vi "Hindbrain.vi"() -> ()   [LabVIEW 2012]
doc: "Hindbrain_RobotBrainExample. This VI is an example of the Hindbrain layer of the Olin Robot Architecture. It collects all SENSE data and sends it up three neural clusters to the Midbrain and accepts one ACT cluster from Midbrain to drive all robot actuators. \nVI also contains a simple robot simulation to allow control code development"
uses:
  GlobalACT.vi
  WindDir.vi
  WindSpeed.vi
  G_Boat Speed.vi
  GlobalWhatAroundMe.vi
  GlobalWhereAmI.vi
  GlobalHowAmI.vi
panel:
  out "WhereSensor":T1
  out "Act Command":cluster{"Velocity":dbl, "Direction":dbl}
  out "Act":bool
  out "How?":bool
  out "What?":bool
  in  "stop":bool
  out "Where":bool
  out "HowAmI?":cluster{"T":dbl, "Battery":dbl, "Temp":dbl}
  out "WhatAroundMe?":cluster{"T":dbl, "Range":dbl, "Bearing":dbl}[](array[cluster])
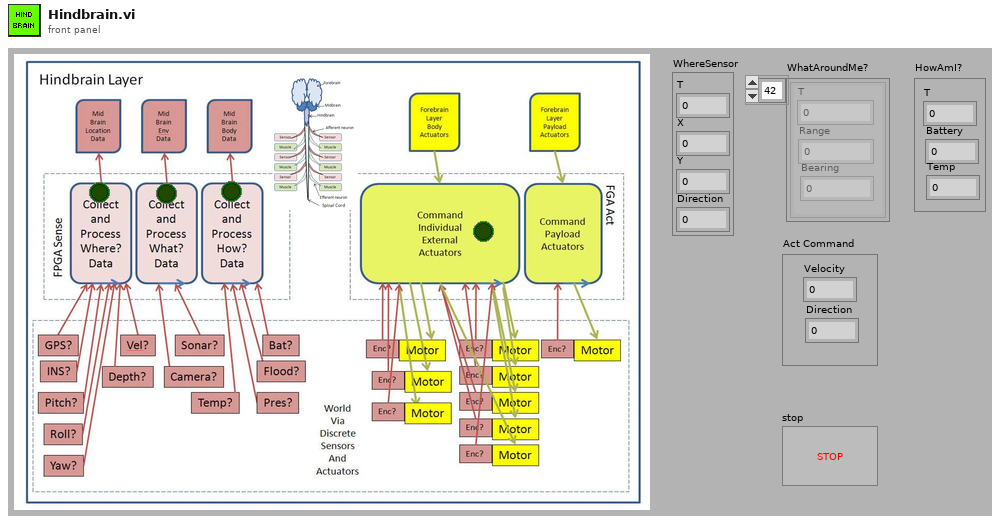
[diagram p1: front panel]
types:
  T1 = cluster{"T":dbl, "X":dbl, "Y":dbl, "Direction":dbl}
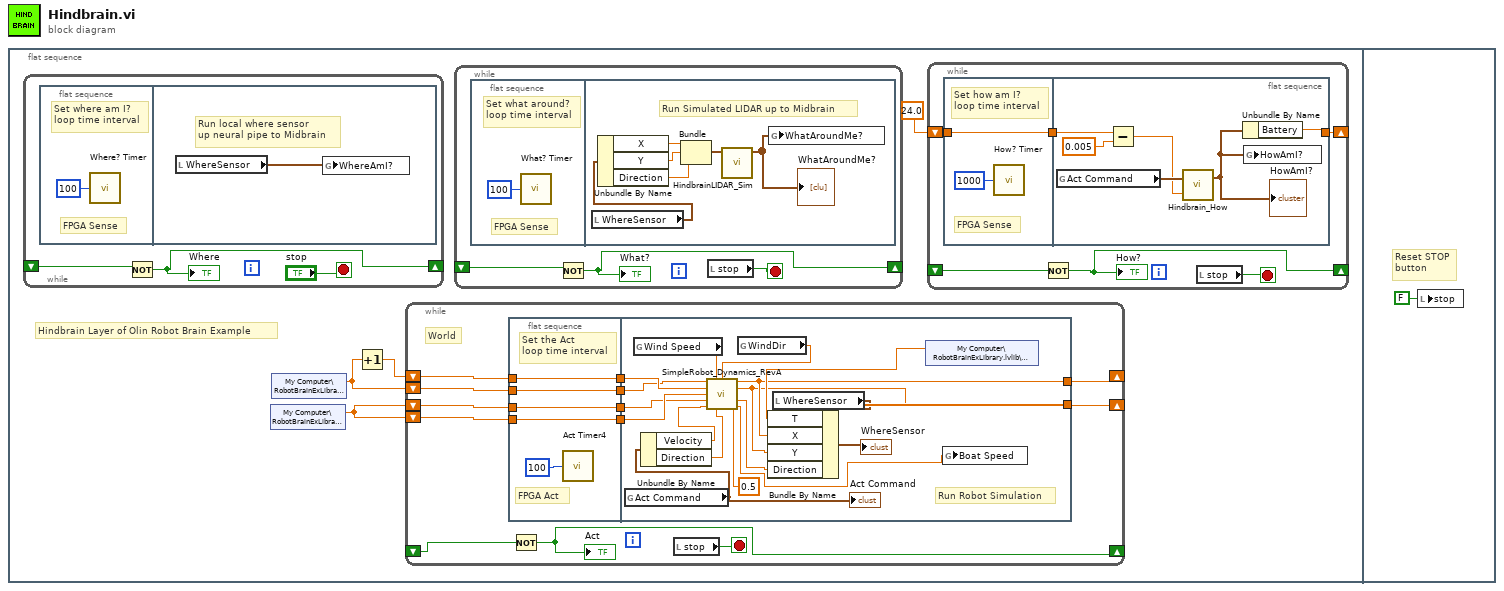
[diagram p0: block diagram]
diagram:
  n1 = flat-sequence {
    frame #0 {
      # "Hindbrain Layer of Olin Robot Brain Example"
      n2 = while {
        shift-right: [w64] -> _
        shift-left: _ -> [w65]
        stop <- "stop" stop-if-true
        n3 = flat-sequence {
          frame #0 {
            # "FPGA Sense"
            # "Set where am I?\nloop time interval"
            n4 = call "Where? Timer"("Count(mSec)"=u32 100) -> ()  [unwired: 1 out]
          }
          frame #1 {
            # "Run local where sensor\nup neural pipe to Midbrain"
            n5 = local read "WhereSensor"() -> (w68:T1)
            n6 = global write "GlobalWhereAmI.vi" "WhereAmI?"(w68) -> ()
          }
        }
        n7 = Not(x=w65) -> (.not. x?=w64:bool)
        "Where" <- w64
      }
      n8 = shared-variable "My Computer\\RobotBrainExLibrary.lvlib\\Ystart"() -> (w3:dbl)  [unwired: 1 in, 1 out]
      n9 = shared-variable "My Computer\\RobotBrainExLibrary.lvlib\\Xstart"() -> (w2:dbl)  [unwired: 1 in, 1 out]
      n10 = Increment(x=w2) -> (x+1=w1:dbl)
      n11 = while {
        shift-right: [w16] -> _
        shift-left: _ -> [w17]
        shift-right: [w6] -> _
        shift-left: w1 -> [w13]
        shift-left: w2 -> [w11]
        shift-right: [w5] -> _
        shift-left: w3 -> [w9]
        shift-left: w3 -> [w7]
        stop <- w15 stop-if-true
        # "World"
        n12 = flat-sequence {
          tunnel: [w21] -> w14
          tunnel: w13 -> [w21]
          tunnel: [w20] -> w12
          tunnel: w11 -> [w20]
          tunnel: [w19] -> w10
          tunnel: w9 -> [w19]
          tunnel: [w18] -> w8
          tunnel: w7 -> [w18]
          tunnel: w14 -> [w29]
          tunnel: [w34] -> w6
          tunnel: w12 -> [w28]
          tunnel: w10 -> [w26]
          tunnel: [w33] -> w5
          tunnel: w8 -> [w27]
          frame #0 {
            # "FPGA Act"
            # "Set the Act\nloop time interval"
            n13 = call "Act Timer4"("Count(mSec)"=u32 100) -> ()  [unwired: 1 out]
          }
          frame #1 {
            # "Run Robot Simulation"
            n14 = global read "GlobalACT.vi" "Act Command"() -> (w39:cluster{"Velocity":dbl, "Direction":dbl})
            "Act Command" <- w39
            n15 = global read "WindSpeed.vi" "Wind Speed"() -> (w25:dbl)
            n16 = Unbundle By Name(w39) -> ("Velocity"=w38:dbl, "Direction"=w37:dbl)
            n17 = global read "WindDir.vi" "WindDir"() -> (w24:dbl)
            n18 = call "SimpleRobot_Dynamics_RevA.vi"("x0"=w28, "Wind Speed"=w25, "Wind Direction"=w24, "x1"=w29, "y0"=w27, "y1"=w26, "Velocity"=w38, "Direction"=w37, "DeltaT (timestep)"=0.5) -> ("x 2"=w34:dbl, "y 2"=w33:dbl, "Direction 2"=w32:dbl, "Boat Velocity Out"=w23:dbl)  [unwired: 3 in]
            n19 = local read "WhereSensor"() -> (w30:T1)
            n20 = shared-variable "My Computer\\RobotBrainExLibrary.lvlib\\MissionTime"() -> (w35:dbl)  [unwired: 1 in, 1 out]
            n21 = Bundle By Name(cluster=w30, "T"=w35, "X"=w34, "Y"=w33, "Direction"=w32) -> (→"WhereSensor":T1)
            n22 = global write "G_Boat Speed.vi" "Boat Speed"(w23) -> ()
          }
        }
        n23 = Not(x=w17) -> (.not. x?=w16:bool)
        "Act" <- w16
        n24 = local read "stop"() -> (w15:bool)
      }
      n25 = while {
        shift-right: [w55] -> _
        shift-left: _ -> [w56]
        stop <- w54 stop-if-true
        n26 = flat-sequence {
          frame #0 {
            # "FPGA Sense"
            # "Set what around?\nloop time interval"
            n27 = call "What? Timer"("Count(mSec)"=u32 100) -> ()  [unwired: 1 out]
          }
          frame #1 {
            # "Run Simulated LIDAR up to Midbrain"
            n28 = local read "WhereSensor"() -> (w62:T1)
            n29 = Unbundle By Name(w62) -> ("X"=w60:dbl, "Y"=w59:dbl, "Direction"=w58:dbl)
            n30 = Bundle("X"=w60, "Y"=w59, "Direction"=w58) -> (w61:cluster{"X":dbl, "Y":dbl, "Direction":dbl})  [unwired: 1 in]
            n31 = call "HindbrainLIDAR_Sim.vi"("SubPosition"=w61) -> ("WhatAroundMe?"=w63:cluster{"T":dbl, "Range":dbl, "Bearing":dbl}[])  [unwired: 10 in]
            "WhatAroundMe?" <- w63
            n32 = global write "GlobalWhatAroundMe.vi" "WhatAroundMe?"(w63) -> ()
          }
        }
        n33 = Not(x=w56) -> (.not. x?=w55:bool)
        "What?" <- w55
        n34 = local read "stop"() -> (w54:bool)
      }
      n35 = while {
        shift-right: [w44] -> _
        shift-left: _ -> [w45]
        shift-right: [w40] -> _
        shift-left: 24.0 -> [w41]
        stop <- w43 stop-if-true
        n36 = flat-sequence {
          tunnel: [w46] -> w42
          tunnel: w41 -> [w46]
          tunnel: w42 -> [w52]
          tunnel: [w48] -> w40
          frame #0 {
            # "FPGA Sense"
            # "Set how am I?\nloop time interval"
            n37 = call "How? Timer"("Count(mSec)"=u32 1000) -> ()  [unwired: 1 out]
          }
          frame #1 {
            n38 = global read "GlobalACT.vi" "Act Command"() -> (w51:cluster{"Velocity":dbl, "Direction":dbl})
            n39 = Subtract(x=w52, y=0.005) -> (x-y=w50:dbl)
            n40 = call "Hindbrain_How.vi"("Battery"=w50, "Act Command"=w51) -> ("HowAmI?"=w49:cluster{"T":dbl, "Battery":dbl, "Temp":dbl})  [unwired: 1 in]
            "HowAmI?" <- w49
            n41 = Unbundle By Name(w49) -> ("Battery"=w48:dbl)
            n42 = global write "GlobalHowAmI.vi" "HowAmI?"(w49) -> ()
          }
        }
        n43 = Not(x=w45) -> (.not. x?=w44:bool)
        "How?" <- w44
        n44 = local read "stop"() -> (w43:bool)
      }
    }
    frame #1 {
      # "Reset STOP\nbutton"
      n45 = local write "stop"(FALSE ("stop")) -> ()
    }
  }
